vi "Drop Waypoint.vi"(1 "TA Speed":dbl, 2 "TA GPS":cluster{"X pos":i32, "Y pos":i32, "Heading":dbl}={"X pos"=250, "Y pos"=250, "Heading"=0.0}, 3 "Our GPS":cluster{"X pos":i32, "Y pos":i32, "Heading":dbl}={"X pos"=250, "Y pos"=250, "Heading"=0.0}) -> (0 "Output Waypoint":T1={"Type"=enum."Start", "X"=250, "Y"=250, "Speed"=0, "Behaviors"=enum."Open Water Transit"})   [LabVIEW 2014]
panel:
  in  "Waypoint seed":T1={"Type"=enum."Start", "X"=250, "Y"=250, "Speed"=0, "Behaviors"=enum."Open Water Transit"}
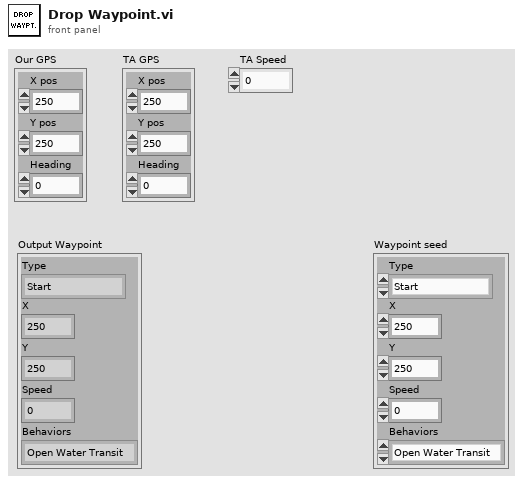
[diagram p1: front panel]
types:
  T1 = cluster{"Type":enum16{"Start", "Waypoint", "End"}, "X":i32, "Y":i32, "Speed":i32, "Behaviors":enum16{"Open Water Transit", "P-Wall Follow", "S-Wall Follow", "Dock", "Chase"}}
  T2 = enum16{"Open Water Transit", "P-Wall Follow", "S-Wall Follow", "Dock", "Chase"}
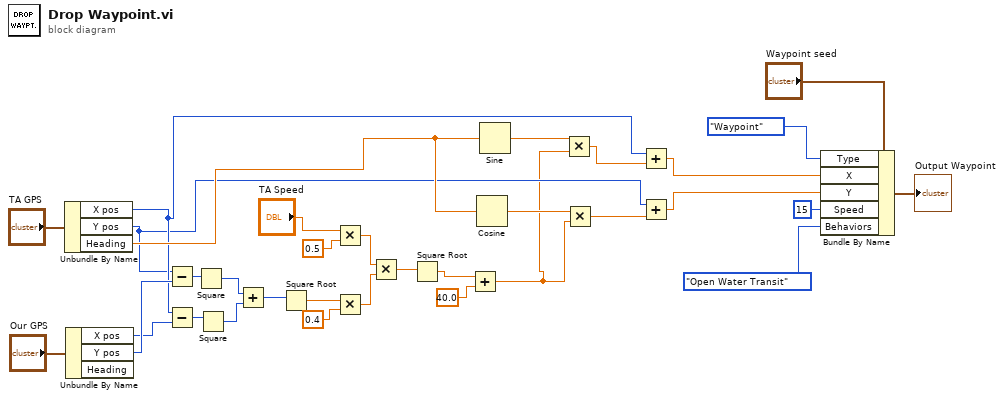
[diagram p0: block diagram]
diagram:
  n1 = Unbundle By Name("TA GPS") -> ("X pos"=w10:i32, "Y pos"=w8:i32, "Heading"=w15:dbl)
  n2 = Unbundle By Name("Our GPS") -> ("X pos"=w26:i32, "Y pos"=w27:i32)  [unwired: 1 out]
  n3 = Subtract(x=w8, y=w27) -> (x-y=w25:i32)
  n4 = Subtract(x=w10, y=w26) -> (x-y=w24:i32)
  n5 = Square(x=w25) -> (x^2=w22:i32)
  n6 = Square(x=w24) -> (x^2=w21:i32)
  n7 = Add(x=w22, y=w21) -> (x+y=w23:i32)
  n8 = Square Root(x=w23) -> (sqrt(x)=w20:dbl)
  n9 = Multiply(x="TA Speed", y=0.5) -> (x*y=w1:dbl)
  n10 = Multiply(x=w20, y=0.4) -> (x*y=w17:dbl)
  n11 = Multiply(x=w1, y=w17) -> (x*y=w4:dbl)
  n12 = Square Root(x=w4) -> (sqrt(x)=w3:dbl)
  n13 = Add(x=w3, y=40.0) -> (x+y=w6:dbl)
  n14 = Cosine(x=w15) -> (cos(x)=w14:dbl)
  n15 = Sine(x=w15) -> (sin(x)=w13:dbl)
  n16 = Multiply(x=w13, y=w6) -> (x*y=w9:dbl)
  n17 = Multiply(x=w14, y=w6) -> (x*y=w7:dbl)
  n18 = Add(x=w10, y=w9) -> (x+y=w11:dbl)
  n19 = Add(x=w8, y=w7) -> (x+y=w12:dbl)
  n20 = Bundle By Name(cluster="Waypoint seed", "Type"=enum16{"Start", "Waypoint", "End"}."Waypoint", "X"=w11, "Y"=w12, "Speed"=15, "Behaviors"=T2."Open Water Transit") -> (→"Output Waypoint":T1)
